vi "Read Aout Limit.vi"(8 "error in (no error)":errorcluster, 11 "VISA resource name":refnum<visa-resource-name>) -> (0 "error out":errorcluster, 2 "aout limit":T1, 3 "VISA resource name out":refnum<visa-resource-name>)   [LabVIEW 2019, in "Andeen-Hagerling 2700A.lvlib"]
doc: "Return the upper and lower protection limits, respectively, of\nthe capacitance and loss channel output voltages in volts.\nThese protection limits apply only to voltage levels produced\nby the deviation subsystem. They do not limit the output\nderived from internal bias voltage sources."
uses:
  Andeen-Hagerling 2700A.lvlib
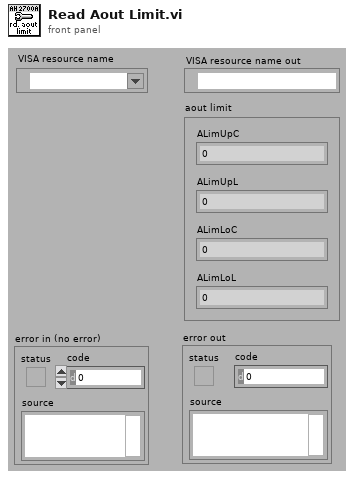
[diagram p1: front panel]
types:
  T1 = cluster{"ALimUpC":dbl, "ALimUpL":dbl, "ALimLoC":dbl, "ALimLoL":dbl}
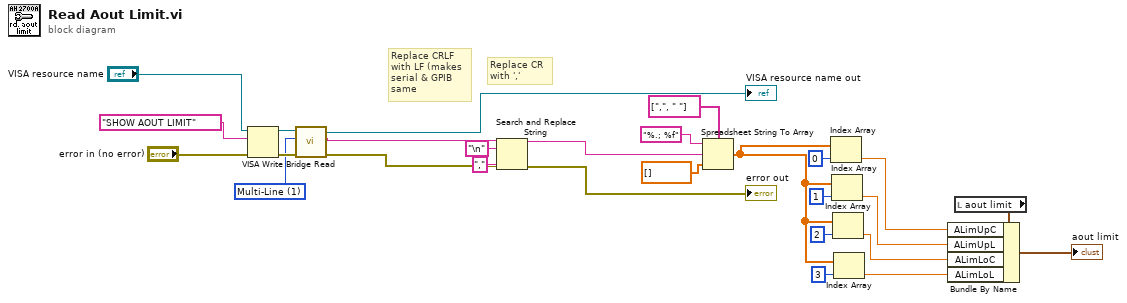
[diagram p0: block diagram]
diagram:
  w3 = u16 1 items=["Single Line", "Multi-Line"] ("Multiline")
  # "Replace CR\nwith ','"
  # "Replace CRLF\nwith LF (makes\nserial & GPIB \nsame"
  n1 = VISA Write(VISA resource name="VISA resource name", write buffer="SHOW AOUT LIMIT" ("command"), error in (no error)="error in (no error)") -> (VISA resource name out=w25:refnum<visa-resource-name>, error out=w24:errorcluster)  [unwired: 1 out]
  n2 = call "Bridge Read.vi"("error in (no error)"=w24, "multiline"=w3, "VISA resource name"=w25) -> ("error out"=w1:errorcluster, "read buffer"=w2:string, "VISA resource name out"=→"VISA resource name out":refnum<visa-resource-name>)  [unwired: 6 in]
  n3 = Search and Replace String(input string=w2, search string="\n", replace string="," ("replace string (\"\")"), error in=w1) -> (result string=w7:string, error out=→"error out":errorcluster)  [unwired: 4 in, 2 out]
  n4 = Spreadsheet String To Array(delimiter (Tab)=string[] [",", " "], format string="%.; %f", spreadsheet string=w7, array type (2D Dbl)=dbl[] []) -> (array=w15:dbl[])
  n5 = Index Array(array=w15, index=0) -> (element=w12:dbl)
  n6 = Index Array(array=w15, index=1) -> (element=w11:dbl)
  n7 = Index Array(array=w15, index=2) -> (element=w10:dbl)
  n8 = Index Array(array=w15, index=3) -> (element=w9:dbl)
  n9 = local read "aout limit"() -> (w13:T1)
  n10 = Bundle By Name(cluster=w13, "ALimUpC"=w12, "ALimUpL"=w11, "ALimLoC"=w10, "ALimLoL"=w9) -> (→"aout limit":T1)
